vi "RSZVB Trace Export Data.vi"(8 "error in (no error)":errorcluster {"code" format="%.0x"}, 9 "File Name (Trc1.s1p)":string="Trc1.s1p", 10 "Trace Name (Trc1)":string="Trc1", 11 "VISA session":refnum<visa-resource-name>) -> (0 "error out":errorcluster {"code" format="%.0x"}, 3 "dup VISA session":refnum<visa-resource-name>)   [LabVIEW 2011]
doc: "This VI stores the trace data of a specified trace to a trace file.\n\nNote(s):\n\nTraces are created using the CALCulte<Ch>:PARameter:SDEFine... command.\n\n*.s<n>p touchstone files (<n> = 2, 3, 4) are intended for a complete set of <n>-port S-parameters. Data export fails if the active channel does not contain the full set of <n>^2 traces. If the necessary trace are available, '<trc_name>' can be the name of any of the traces.\n\nRemote-control command(s):\nMMEMory:STORe:TRACe '<trc_name>','<file_name>'"
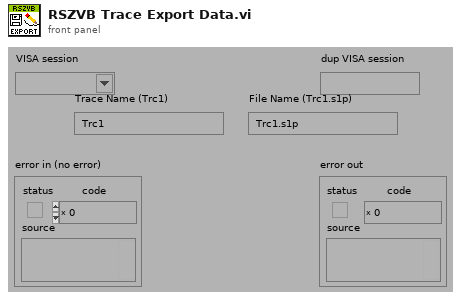
[diagram p1: front panel]
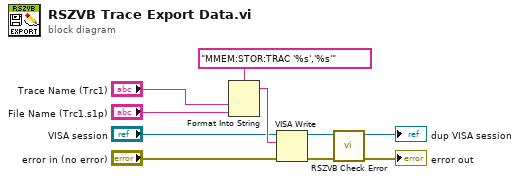
[diagram p0: block diagram]
diagram:
  n1 = Format Into String(format string="MMEM:STOR:TRAC '%s','%s'", "Trace Name (Trc1)", "File Name (Trc1.s1p)") -> (resulting string=w7:string)  [unwired: 2 in, 1 out]
  n2 = VISA Write(VISA resource name="VISA session", write buffer=w7, error in (no error)="error in (no error)") -> (VISA resource name out=w8:refnum<visa-resource-name>, error out=w9:errorcluster)  [unwired: 1 out]
  n3 = call "RSZVB Check Error.vi"("error in (no error)"=w9, "VISA session"=w8) -> ("error out"=→"error out":errorcluster, "dup VISA session"=→"dup VISA session":refnum<visa-resource-name>)  [unwired: 8 in]
